vi "Tool Relay State Initialized.vi"(1 "Action(GET)":enum16{"GET", "SET"}(ring), 5 "Relay 1 Initialized":bool, 7 "Relay 2 Initialized":bool, 11 "error in (no error)":errorcluster) -> (6 "Relay 1 Initialized out":bool, 8 "Relay 2 Initialized out":bool, 15 "error out":errorcluster)   [LabVIEW 2011]
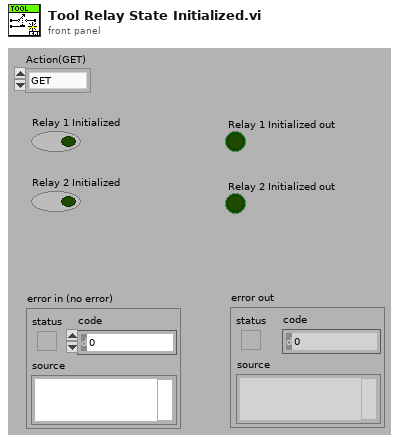
[diagram p1: front panel]
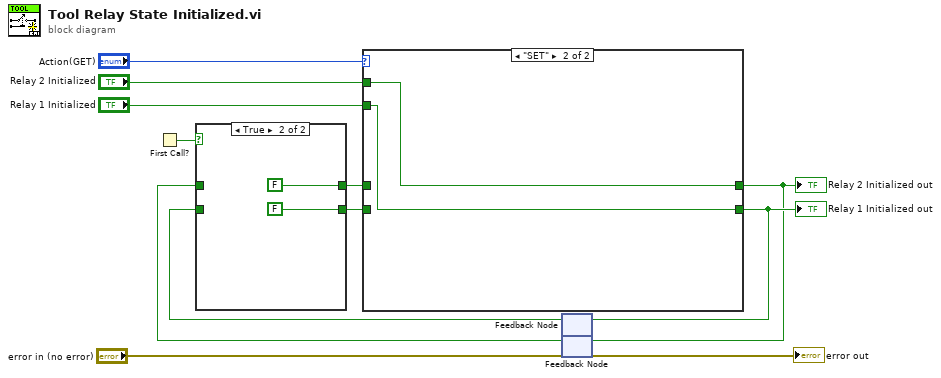
[diagram p0: block diagram]
diagram:
  n1 = First Call?() -> (First Call?: T/F=w8:bool)
  n2 = feedback #1() -> (w9:bool)  [unwired: 1 in]
  n3 = feedback #2() -> (w1:bool)  [unwired: 1 in]
  n4 = case shown="True" w8 {
    tunnel: w9 -> [w13 _]
    tunnel: [w13 FALSE] -> w6
    tunnel: [w12 FALSE] -> w3
    tunnel: w1 -> [w12 _]
    frame False {
    }
    frame True {
    }
  }
  n5 = case shown="\"SET\"" "Action(GET)" {
    tunnel: [w17 w19] -> w7
    tunnel: w6 -> [w17 _]
    tunnel: "Relay 1 Initialized" -> [_ w19]
    tunnel: "Relay 2 Initialized" -> [_ w18]
    tunnel: [w16 w18] -> w2
    tunnel: w3 -> [w16 _]
    frame "GET", Default {
    }
    frame "SET" {
    }
  }
  "Relay 1 Initialized out" <- w7
  "Relay 2 Initialized out" <- w2
  n6 = feedback-in #1(w7) -> ()
  n7 = feedback-in #2(w2) -> ()
  "error out" <- "error in (no error)"
